vi "Error Query.vi"(8 "error in (no error)":errorcluster, 11 "VISA resource name":refnum<visa-resource-name>) -> (0 "error out":errorcluster, 1 "Fault Value":string, 2 "Error Value":string, 3 "VISA resource name out":refnum<visa-resource-name>)   [LabVIEW 2021, in "Sorensen M9A Series.lvlib"]
doc: "This VI provides very basic error checking for a Sorensen power supply. The VI only checks to see if either a fault (FAULT?) or error (ERR?) has occured."
uses:
  Sorensen M9A Series.lvlib
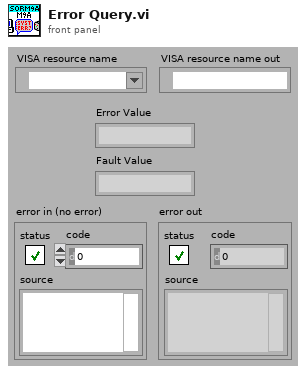
[diagram p1: front panel]
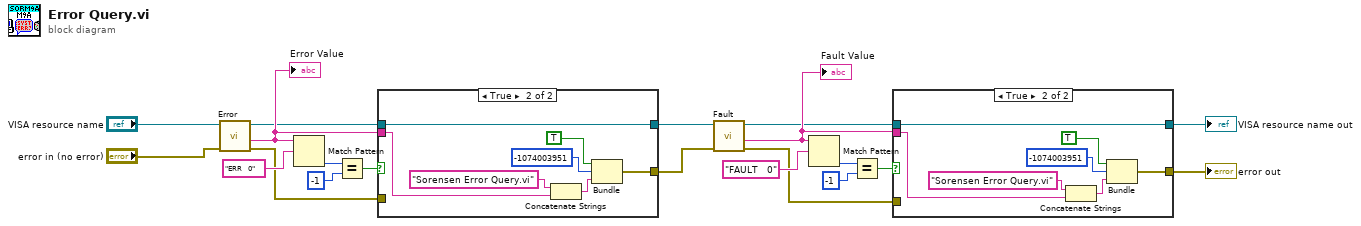
[diagram p0: block diagram]
diagram:
  n1 = call "Error.vi"("error in (no error)"="error in (no error)", "VISA resource name"="VISA resource name") -> ("error out"=w8:errorcluster, "Error Value (string)"=w7:string, "VISA resource name out"=w6:refnum<visa-resource-name>)  [unwired: 6 in, 1 out]
  "Error Value" <- w7
  n2 = Match Pattern(string=w7, regular expression="ERR   0") -> (offset past match=w19:i32)  [unwired: 1 in, 3 out]
  n3 = Equal?(x=w19, y=-1) -> (x = y?=w17:bool)
  n4 = case shown="True" w17 {
    tunnel: w6 -> [w22 w26]
    tunnel: w8 -> [w21 _]
    tunnel: [w21 w27] -> w4
    tunnel: [w22 w26] -> w5
    tunnel: w7 -> [_ w24]
    frame False {
    }
    frame True {
      n5 = Concatenate Strings("Sorensen Error Query.vi", w24) -> (w25:string)
      n6 = Bundle(TRUE, -1074003951, w25) -> (w27:errorcluster)  [unwired: 1 in]
    }
  }
  n7 = call "Fault.vi"("error in (no error)"=w4, "VISA resource name"=w5) -> ("error out"=w3:errorcluster, "Fault Value (string)"=w2:string, "VISA resource name out"=w1:refnum<visa-resource-name>)  [unwired: 6 in, 1 out]
  "Fault Value" <- w2
  n8 = Match Pattern(string=w2, regular expression="FAULT   0") -> (offset past match=w16:i32)  [unwired: 1 in, 3 out]
  n9 = Equal?(x=w16, y=-1) -> (x = y?=w13:bool)
  n10 = case shown="True" w13 {
    tunnel: [w31 w36] -> w11
    tunnel: w3 -> [w31 _]
    tunnel: w1 -> [w30 w35]
    tunnel: [w30 w35] -> w12
    tunnel: w2 -> [_ w33]
    frame False {
    }
    frame True {
      n11 = Concatenate Strings("Sorensen Error Query.vi", w33) -> (w32:string)
      n12 = Bundle(TRUE, -1074003951, w32) -> (w36:errorcluster)  [unwired: 1 in]
    }
  }
  "VISA resource name out" <- w12
  "error out" <- w11
